vi "Initialize.vi"(8 "error in (no error)":errorcluster, 11 "Laser_Oxxius in":refnum<class "Laser_Oxxius.lvclass">) -> (0 "error out":errorcluster, 3 "Laser_Oxxius out":refnum<class "Laser_Oxxius.lvclass">)   [LabVIEW 2020, in "Laser_Oxxius.lvlib" / "Laser_Oxxius.lvclass"]
uses:
  Laser_Oxxius.lvclass
  E:/Development/DevHardSoftware/MMicroscopy/HardwareAdapter/Lasers/Dependencies/Oxxius_Boxx.dll
  MMicroscopy/HardwareAdapter/Lasers/Dependencies/Oxxius_Boxx.dll
  Laser_Oxxius.lvclass/Laser_Oxxius.ctl
  HAL Layer/Component/Laser/Laser/Laser.lvclass
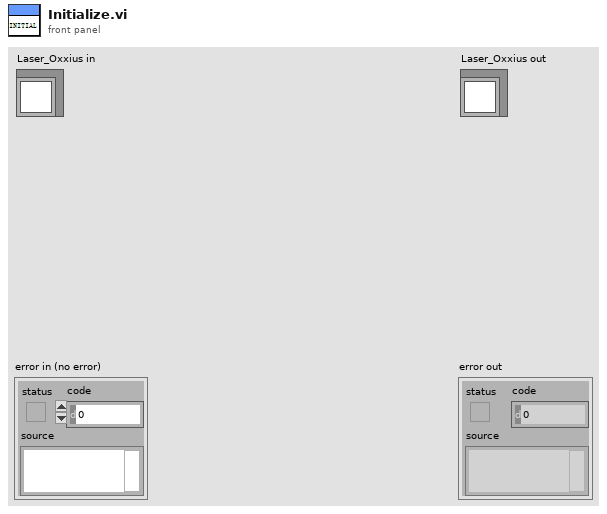
[diagram p1: front panel]
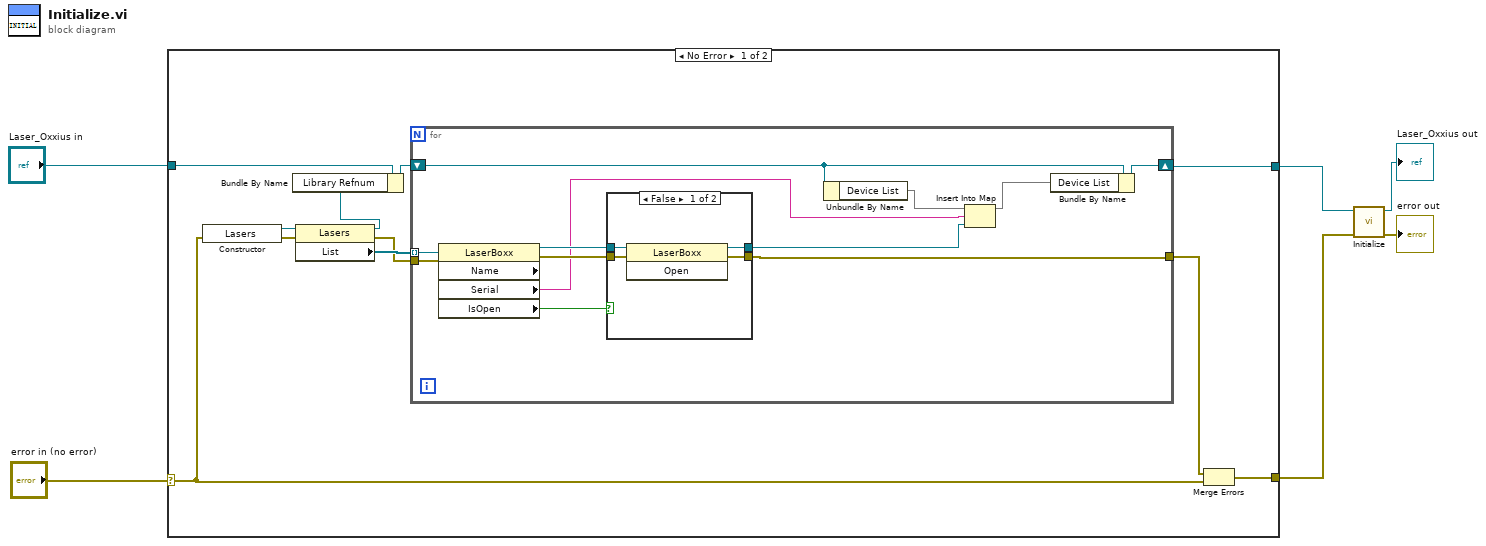
[diagram p0: block diagram]
diagram:
  n1 = case shown="No Error" "error in (no error)" {
    selector: "error in (no error)" -> [w10 w37]
    tunnel: [w17 w37] -> w4
    tunnel: [w11 w36] -> w2
    tunnel: "Laser_Oxxius in" -> [w9 w36]
    frame No Error {
      n2 = constructor class="Lasers"(error in=w10) -> (reference out=w15:refnum<k24>, error out=w14:errorcluster)  [unwired: 2 in, 1 out]
      n3 = property class="Lasers"(reference=w15, error in=w14) -> (reference out=w7:refnum<k24>, error out=w13:errorcluster, "List"=w16:refnum<k24>[])
      n4 = Bundle By Name(cluster=w9, "Library Refnum"=w7) -> (w8:refnum<class "Laser_Oxxius.lvclass">)
      n5 = for {
        tunnel: w16 -> [w29] mode=indexing
        tunnel: w13 -> [w28]
        tunnel: [w27] -> w12
        shift-right: [w23] -> w11
        shift-left: w8 -> [w22]
        n6 = property class="LaserBoxx" props=["Name", "Serial", "IsOpen"](reference=w29, error in=w28) -> (reference out=w26:refnum<k24>, error out=w25:errorcluster, "Serial"=w20:string, "IsOpen"=w24:bool)  [unwired: 1 out]
        n7 = case shown="False" w24 {
          tunnel: w25 -> [w33 w35]
          tunnel: w26 -> [w32 w34]
          tunnel: [w31 w35] -> w27
          tunnel: [w30 w34] -> w19
          frame False {
            n8 = invoke class="LaserBoxx" method="Open"(reference=w32, error in=w33) -> (reference out=w30:refnum<k24>, error out=w31:errorcluster)  [unwired: 1 in, 1 out]
          }
          frame True {
          }
        }
        n9 = Unbundle By Name(w22) -> ("Device List"=w21:map{string, refnum<k24>})
        n10 = Insert Into Map(map in=w21, key=w20, value=w19) -> (map out=w18:map{string, refnum<k24>})  [unwired: 2 out]
        n11 = Bundle By Name(cluster=w22, "Device List"=w18) -> (w23:refnum<class "Laser_Oxxius.lvclass">)
      }
      n12 = Merge Errors(w12, w10) -> (w17:errorcluster)
    }
    frame Error {
    }
  }
  n13 = call-parent "Initialize.vi"("error in (no error)"=w4, "Device in"=w2) -> ("error out"=→"error out":errorcluster, "Device out"=→"Laser_Oxxius out":refnum<class "Laser_Oxxius.lvclass">)  [unwired: 8 in]
